vi "CC Set Filter Strings.vi"(8 "error in (no error)":errorcluster, 10 "Strings":string[](array[string]), 11 "refs":refnum<vi>[](array[refnum])) -> (0 "error out":errorcluster)   [LabVIEW 2024]
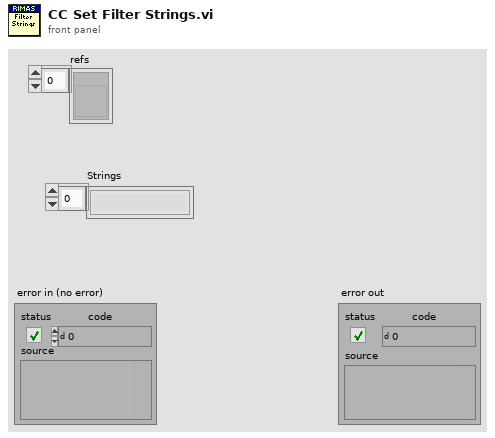
[diagram p1: front panel]
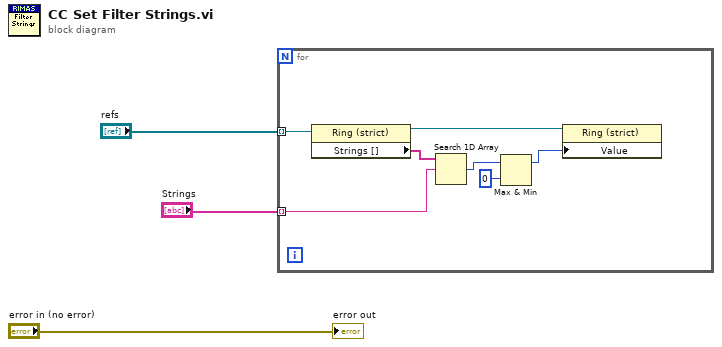
[diagram p0: block diagram]
diagram:
  n1 = for {
    tunnel: "refs" -> [w10] mode=indexing
    tunnel: "Strings" -> [w6] mode=indexing
    n2 = property class="Ring (strict)"(reference=w10) -> (reference out=w5:refnum<vi>, "Strings []"=w7:string[])  [unwired: 1 in, 1 out]
    n3 = Search 1D Array(1D array=w7, element=w6) -> (index of element=w8:i32)  [unwired: 1 in]
    n4 = Max & Min(x=w8, y=0) -> (max(x,y)=w4:i32)  [unwired: 1 out]
    n5 = property class="Ring (strict)"(reference=w5, "Value"=w4) -> ()  [unwired: 1 in, 2 out]
  }
  "error out" <- "error in (no error)"
